vi "StopButton.vi"(11 "String":string) -> (3 "Enum":enum16{"Ok", "Cancel", "Timeout"}(ring))   [LabVIEW 2020]
panel:
  in  "Cancel Button":bool
  in  "OK Button":bool
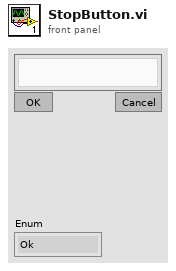
[diagram p1: front panel]
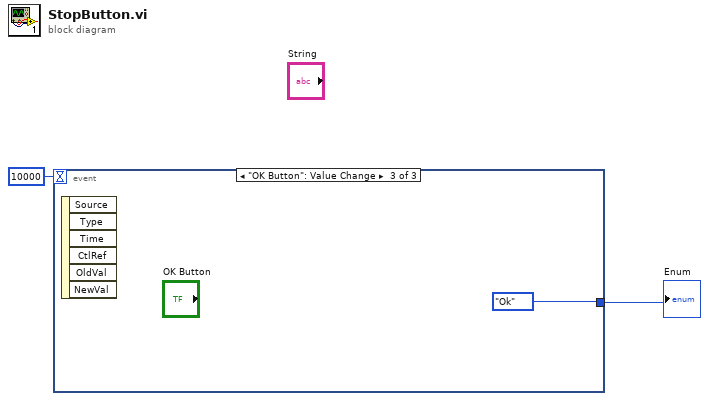
[diagram p0: block diagram]
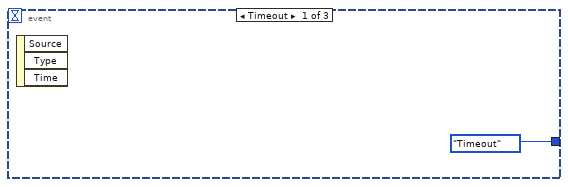
[diagram p2: hidden frame]
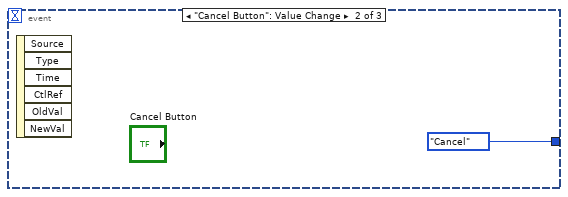
[diagram p3: hidden frame]
diagram:
  n1 = event shown="[2] \"OK Button\": Value Change" {
    selector: _ -> [_ _ _]
    dyn-events: _ -> [_ _ _]
    timeout: 10000 -> [_ _ _]
    tunnel: [enum16{"Ok", "Cancel", "Timeout"}."Timeout" enum16{"Ok", "Cancel", "Timeout"}."Cancel" enum16{"Ok", "Cancel", "Timeout"}."Ok"] -> w1
    event Timeout {
      n2 = event-data() -> ()  [unwired: 1 in, 3 out]
    }
    event "Cancel Button": Value Change {
      n3 = event-data() -> ()  [unwired: 1 in, 6 out]
    }
    event "OK Button": Value Change {
      n4 = event-data() -> ()  [unwired: 1 in, 6 out]
    }
  }
  "Enum" <- w1
